vi "Read PIDDIDs.vi"(4 "Type":T1, 6 "Diagnostic Protocol":T4, 7 "ID":u16, 8 "error in (no error)":errorcluster, 9 "Lookup":variant, 10 "Values in":dbl[](array[numeric]), 11 "ADCS Connection":T2) -> (0 "error out":errorcluster, 1 "success?":bool, 2 "Values out":dbl[](array[numeric]), 3 "diag ref out":T2, 5 "data out":u8[](array[numeric]))   [LabVIEW 2015, in "Diagnostics Addon Engine.lvlib"]
uses:
  Diagnostics Addon Engine.lvlib
  <vilib>/Automotive Diagnostic Command Set/Diagnostic Transport.llb/Diag Reference.ctl
  <vilib>/Automotive Diagnostic Command Set/Diagnostic Transport.llb/Transport Protocol Selector.ctl
  <vilib>/Automotive Diagnostic Command Set/Diagnostic Transport.llb/Diag CAN Frame Log.ctl
  Shared/Types/Diagnostic Protocols.ctl
  Shared/Types/MessageType Selector.ctl
  Initialize Raw XNET Frame.vi
  <vilib>/xnet/xnet.llb/XNET Convert.vi
  <vilib>/xnet/xnet.llb/XNET Convert (Frame Raw to Signal).vi
  <vilib>/NI Veristand/Custom Device Tools/Custom Device Utility Library/NI VeriStand - Print Debug String.vi
  Convert ID to Raw Data.vi
  Shared/SubVIs/GUID Lookup.vi
  <vilib>/Automotive Diagnostic Command Set/Diagnostic Transport.llb/Apply Success Failure Error.vi
  <vilib>/Automotive Diagnostic Command Set/Diagnostic Transport.llb/Diagnostic Service.vi
  GMLAN/GMLAN.lvlib
  <vilib>/addons/Automotive Diagnostic Command Set/NI_Automotive Diagnostic Command Set.lvlib
  Shared/Diagnostics Addon Shared.lvlib
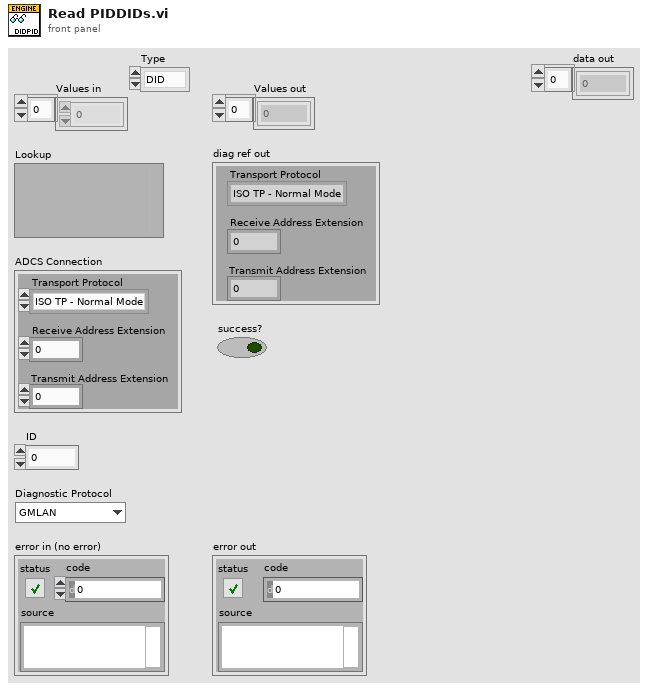
[diagram p1: front panel]
types:
  T1 = typedef "Diagnostics Addon Shared.lvlib/MessageType Selector.ctl" = enum16{"DID", "PID", "CPID", "Write Memory", "Read Memory", "DTC Control", "IO Cmd", "IO Resp", "Routine Start Cmd", "Routine Start Resp", "Routine Status Cmd", "Routine Status Resp", "Routine Stop Cmd", "Routine Stop Resp"}
  T2 = typedef "NI_Automotive Diagnostic Command Set.lvlib/Diag Reference.ctl" = cluster{"Diag CAN Handle":u32, "Transport Protocol":T3, "Receive Address Extension":u8, "Transmit Address Extension":u8, "Receive CAN Id":u32, "Transmit CAN Id":u32, "Diag CAN Queue":refnum<queue>, "Log Frames ?":bool, "My TP Address":u8, "Other TP Address":u8, "T1":u16, "T2":u16, "T3":u16, "T4":u16, "Tx SN":u8, "Block Size":u8, "Rx SN":u8, "VW TP Initialized?":bool, "Tx block no":u8, "baud rate":u32, "Interface":string, "Channel Diag CAN Handle":u32, "UDP Connection ID":refnum<k16>, "TCP Connection ID":refnum<k5>, "Target IP Addr":u32, "Source Address":u16, "Target Address":u16, "Send Header NACK?":bool, "DLL Handle":u32, "NAD":u8, "Time Stamp read first":dbl, "Time Stamp read last":dbl, "Time Stamp write first":dbl, "Time Stamp write last":dbl, "Time Stamp write":dbl, "Time Stamp read":dbl}
  T3 = typedef "NI_Automotive Diagnostic Command Set.lvlib/Transport Protocol Selector.ctl" = enum16{"ISO TP - Normal Mode", "ISO TP - Mixed Mode", "VW TP 2.0", "Diagnostics on IP", "ISO TP LIN"}
  T4 = typedef "Diagnostics Addon Shared.lvlib/Diagnostic Protocols.ctl" = enum16{"GMLAN", "KWP-2000", "UDS"}
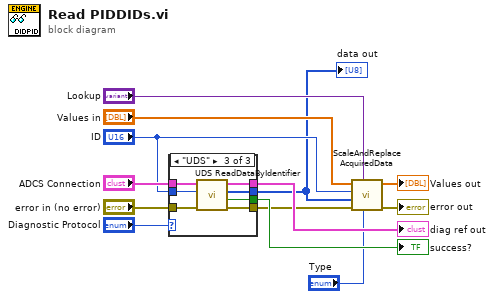
[diagram p0: block diagram]
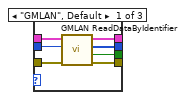
[diagram p2: hidden frame]
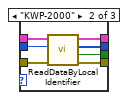
[diagram p3: hidden frame]
diagram:
  n1 = case shown="\"UDS\"" "Diagnostic Protocol" {
    tunnel: "error in (no error)" -> [w17 w25 w34]
    tunnel: "ADCS Connection" -> [w19 w27 w33]
    tunnel: [w15 w24 w32] -> w9
    tunnel: [w20 w23 w31] -> w10
    tunnel: [w14 w22 w30] -> w2
    tunnel: "ID" -> [w16 w26 w29]
    tunnel: [w18 w21 w28] -> w13
    frame "GMLAN", Default {
      n2 = call "GMLAN ReadDataByIdentifier.vi"("error in (no error)"=w17, "Data ID (DID)"=w16, "diag ref in"=w19) -> ("error out"=w15:errorcluster, "success?"=w20:bool, "data out"=w14:u8[], "diag ref out"=w18:T2)  [unwired: 5 in]
    }
    frame "KWP-2000" {
      n3 = call <vilib>:"ReadDataByLocalIdentifier.vi"("error in (no error)"=w25, "local ID"=w26, "diag ref in"=w27) -> ("error out"=w24:errorcluster, "success?"=w23:bool, "data out"=w22:u8[], "diag ref out"=w21:T2)  [unwired: 5 in]
    }
    frame "UDS" {
      n4 = call <vilib>:"UDS ReadDataByIdentifier.vi"("error in (no error)"=w34, "ID"=w29, "diag ref in"=w33) -> ("error out"=w32:errorcluster, "success?"=w31:bool, "data out"=w30:u8[], "diag ref out"=w28:T2)  [unwired: 5 in]
    }
  }
  "diag ref out" <- w13
  "success?" <- w10
  "data out" <- w2
  n5 = call "ScaleAndReplaceAcquiredData.vi"("Type"="Type", "Lookup"="Lookup", "error in (no error)"=w9, "Unscaled Data"=w2, "ID"="ID", "VS Data"="Values in") -> ("error out"=→"error out":errorcluster, "VS Data"=→"Values out":dbl[])  [unwired: 4 in]
